vi "Schedule Control.vi"(10 "Schedule Data":T1, 11 "Mode":enum16{"Get", "Set"}(ring)) -> (2 "Schedule Data Out":T1)   [LabVIEW 2013]
uses:
  Schedule Data.ctl
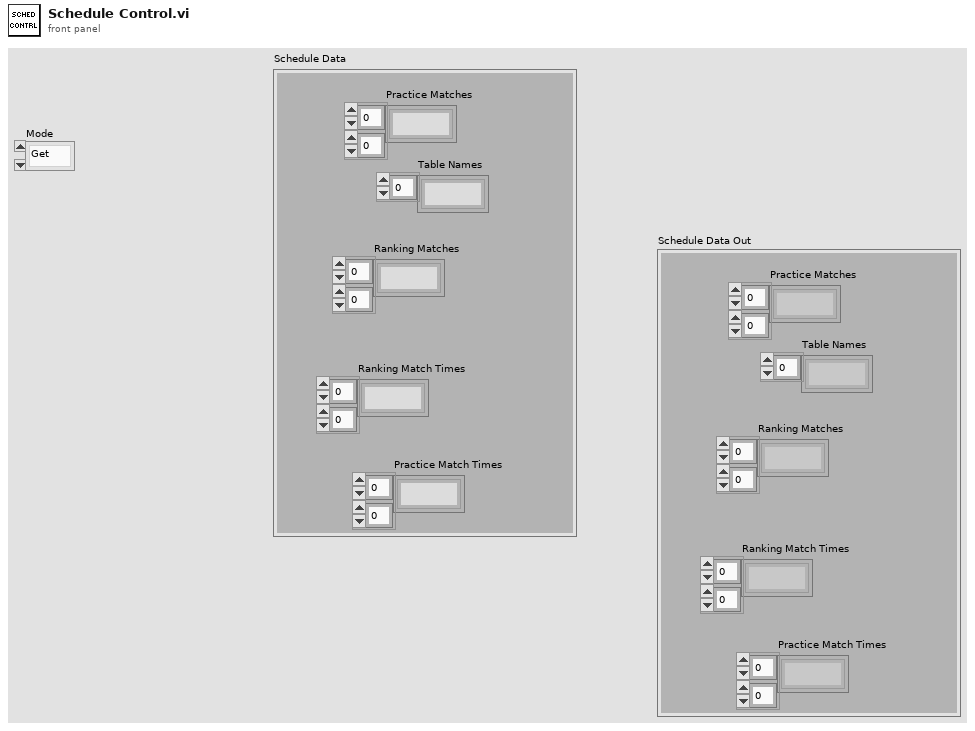
[diagram p1: front panel]
types:
  T1 = typedef "Schedule Data.ctl" = cluster{"Practice Matches":string[][], "Ranking Matches":string[][], "Table Names":string[], "Ranking Match Times":string[][], "Practice Match Times":string[][]}
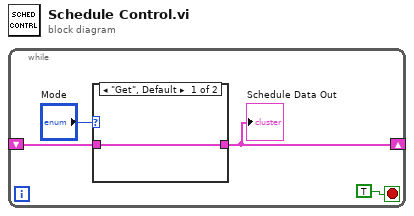
[diagram p0: block diagram]
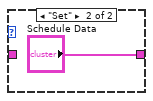
[diagram p2: hidden frame]
diagram:
  n1 = while {
    shift-right: [w2] -> _
    shift-left: _ -> [w1]
    stop <- TRUE stop-if-true
    n2 = case shown="\"Get\", Default" "Mode" {
      tunnel: [w5 "Schedule Data"] -> w2
      tunnel: w1 -> [w5 _]
      frame "Get", Default {
      }
      frame "Set" {
      }
    }
    "Schedule Data Out" <- w2
  }
